vi "Setup7002.vi"(8 "error in":T1, 11 "GPIB IN":string) -> (0 "error out":T1, 3 "GPIB OUT":string)   [LabVIEW 2018]
uses:
  <instrlib>/ke7002/KE7002.LLB/Keith 7002 Open/Close Chan.vi
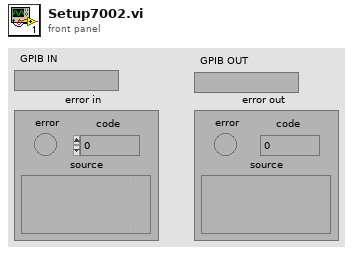
[diagram p1: front panel]
types:
  T1 = cluster{"error":bool, "code":i32, "source":string}
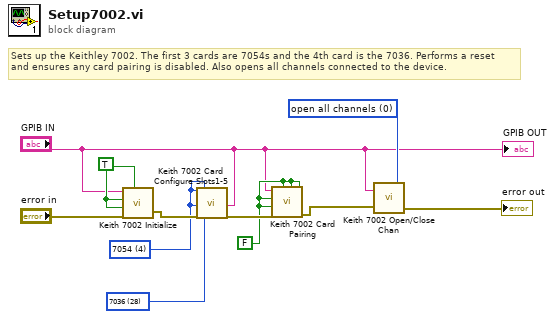
[diagram p0: block diagram]
diagram:
  w4 = u16 0 items=["open all channels", "open channels in channel list", "close channels in channel list"] ("open/close (open all:0)")
  w6 = u16 28 items=["default", "none", "7052", "7053", "7054", "7056", "7057", "7058", "7059", "7061", "7062", "7063", "7064", "7065", "7066", "7067", "7152", "7153", "7154", "7156", "7158", "7164", "7166", "7168", "7169", "7402", "9990", "9991", "7036"] ("slot 4 card type (default:0)")
  w7 = u16 4 items=["default", "none", "7052", "7053", "7054", "7056", "7057", "7058", "7059", "7061", "7062", "7063", "7064", "7065", "7066", "7067", "7152", "7153", "7154", "7156", "7158", "7164", "7166", "7168", "7169", "7402", "9990", "9991"] ("slot 1 card type (default:0)")
  w8 = FALSE ("card pairing slot 2->7")
  w11 = TRUE ("error query")
  # "Sets up the Keithley 7002. The first 3 cards are 7054s and the 4th card is the 7036. Performs a reset\nand ensures any card pairing is disabled. Also opens all channels connected to the device."
  n1 = call <instrlib>:"Keith 7002 Initialize.vi"("GPIB address in"="GPIB IN", "ID query"=w11, "reset"=w11, "error in"="error in", "error query"=w11) -> ("error out"=w10:T1)  [unwired: 1 out]
  n2 = call <instrlib>:"Keith 7002 Card Configure Slots1-5.vi"("slot 1 card type (default:0)"=w7, "slot 2 card type (default:0)"=w7, "error in"=w10, "slot 3 card type (default:0)"=w7, "slot 4 card type (default:0)"=w6, "GPIB address"="GPIB IN") -> ("error out"=w9:T1)  [unwired: 13 in]
  n3 = call <instrlib>:"Keith 7002 Card Pairing.vi"("card pairing slot 3->8"=w8, "card pairing slot 5->10"=w8, "card pairing slot 4->9"=w8, "error in"=w9, "card pairing slot 2->7"=w8, "card pairing slot 1->6"=w8, "GPIB address"="GPIB IN") -> ("error out"=w3:T1)  [unwired: 2 in]
  n4 = call "Keith 7002 Open/Close Chan.vi"("GPIB address"="GPIB IN", "error in"=w3, "open/close (open all:0)"=w4) -> ("error out"=→"error out":T1)  [unwired: 1 in]
  "GPIB OUT" <- "GPIB IN"
